vi "pinMode.vi"(8 "Error In":errorcluster, 10 "Pin Direction":T1, 11 "pin":T2 items=["D0", "D1", "D2", "D3", "D4", "D5", "D6", "D7", "D8", "D9", "D10", "D11", "D12", "D13", "D14", "D15"]) -> (0 "Error Out":errorcluster, 3 "resulting string":string)   [LabVIEW 2014]
uses:
  ctl/digitalPin.ctl
  ctl/pinDirection.ctl
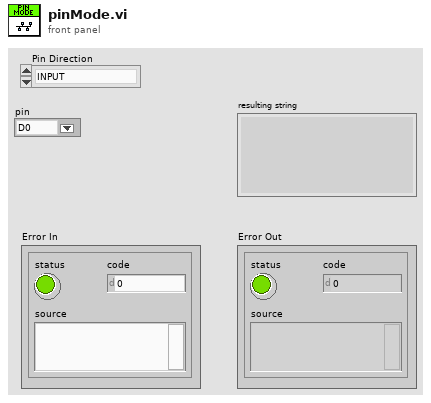
[diagram p1: front panel]
types:
  T1 = typedef "pinDirection.ctl" = enum16{"INPUT", "OUTPUT"}
  T2 = typedef "digitalPin.ctl" = u16
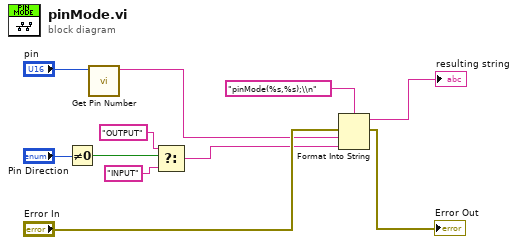
[diagram p0: block diagram]
diagram:
  n1 = Not Equal To 0?(x="Pin Direction") -> (x != 0?=w3:bool)
  n2 = call "Get Pin Number.vi"("pin number"="pin") -> ("String"=w1:string)  [unwired: 10 in]
  n3 = Select(t="OUTPUT", s=w3, f="INPUT") -> (s? t:f=w7:string)
  n4 = Format Into String(format string="pinMode(%s,%s);\\n", error in="Error In", w1, w7) -> (resulting string=→"resulting string":string, error out=→"Error Out":errorcluster)  [unwired: 1 in]
